vi "Untitled 6 (SubVI).vi"(11 "Array":cluster{dbl[], dbl[]}[](array[cluster])) -> (3 "A vs B":cluster{dbl[], dbl[]}[](graph))   [LabVIEW 2016]
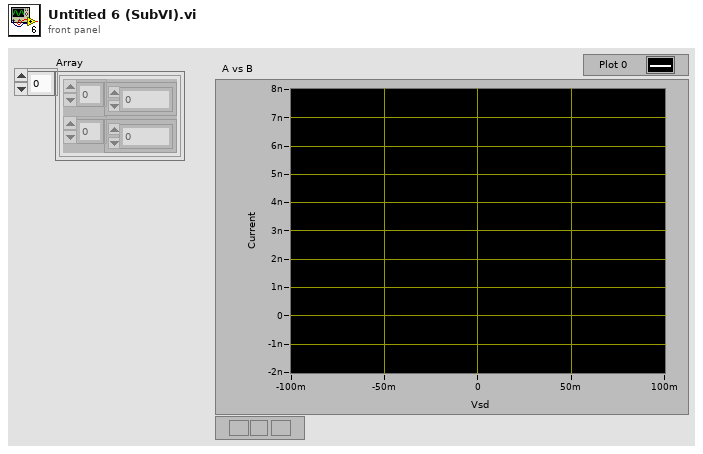
[diagram p1: front panel]
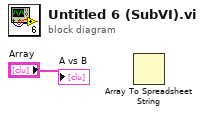
[diagram p0: block diagram]
diagram:
  n1 = Array To Spreadsheet String() -> ()  [unwired: 3 in, 1 out]
  "A vs B" <- "Array"
